vi "Arduino Stepper Driver XY subVI resetPosition.vi"(8 "error in (no error)":errorcluster, 11 "VISA resource name":refnum<visa-resource-name>) -> (0 "error out":errorcluster, 1 "Vertical driver position":i32, 2 "Horizontal driver position":i32, 3 "VISA resource name out":refnum<visa-resource-name>)   [LabVIEW 2013]
panel:
  out "return count":u32
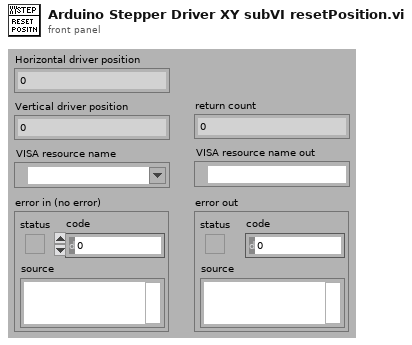
[diagram p1: front panel]
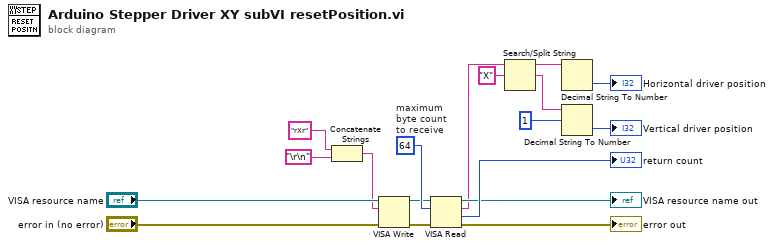
[diagram p0: block diagram]
diagram:
  w13 = u32 64  # maximum byte count to receive
  n1 = Concatenate Strings("rXr" ("string"), "\r\n") -> (w11:string)
  n2 = VISA Write(VISA resource name="VISA resource name", write buffer=w11, error in (no error)="error in (no error)") -> (VISA resource name out=w10:refnum<visa-resource-name>, error out=w9:errorcluster)  [unwired: 1 out]
  n3 = VISA Read(VISA resource name=w10, byte count=w13, error in (no error)=w9) -> (VISA resource name out=→"VISA resource name out":refnum<visa-resource-name>, read buffer=w1:string, return count=→"return count":u32, error out=→"error out":errorcluster)
  n4 = Search/Split String(string=w1, search string/char (-)="X") -> (substring before match=w4:string, match + rest of string=w2:string)  [unwired: 1 in, 1 out]
  n5 = Decimal String To Number(string=w4) -> (number=→"Horizontal driver position":i32)  [unwired: 2 in, 1 out]
  n6 = Decimal String To Number(string=w2, offset=1 ("offset (0)")) -> (number=→"Vertical driver position":i32)  [unwired: 1 in, 1 out]
